vi "ResetHint.vi"(8 "No Error":errorcluster, 11 "Hint Name":T1) -> (0 "error out":errorcluster)   [LabVIEW 2024, in "SDL3.lvlib" / "Hints.lvlib"]
doc: "<B>Summary</B>\nReset a hint to the default value.\n\n<B>Remarks</B>\nThis will reset a hint to the value of the environment variable, or NULL if the environment isn't set. Callbacks will be called normally with this change."
uses:
  Hints.lvlib
  Lib/SDL3.dll
  HintName--combobox.ctl
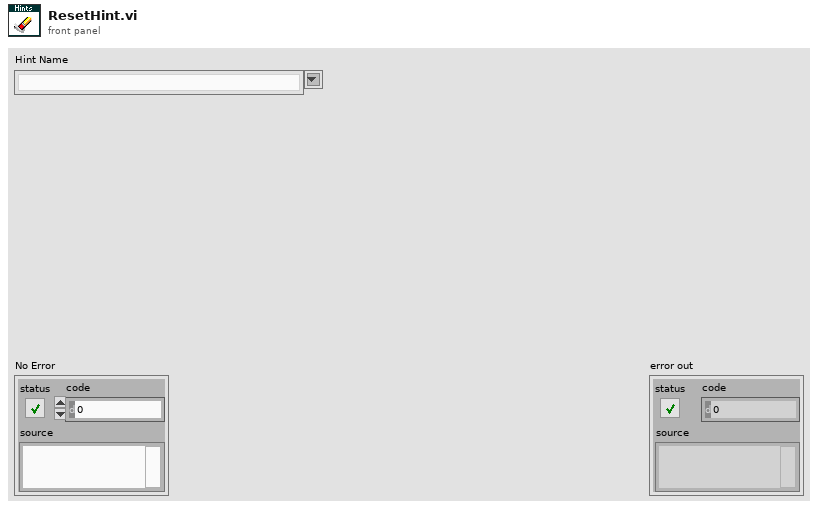
[diagram p1: front panel]
types:
  T1 = typedef "SDL3.lvlib/Hints.lvlib/HintName--combobox.ctl" = string
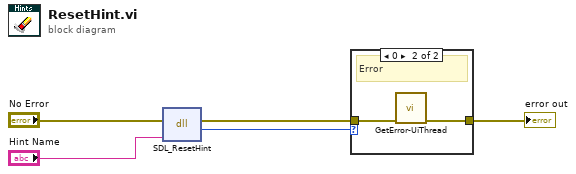
[diagram p0: block diagram]
diagram:
  n1 = dll-call lib="C:/Users/Thomas/Documents/Projects/LV-SDL3/Sources/SDL3/Lib/SDL3.*" fn="SDL_ResetHint"(error in="No Error", "name"="Hint Name") -> (error out=w3:errorcluster, "return type"=w1:i32)  [unwired: 3 in, 1 out]
  n2 = case shown="0" w1 {
    tunnel: w3 -> [w6 w8]
    tunnel: [w6 w7] -> w2
    frame Default {
      # "Ok"
    }
    frame 0 {
      # "Error"
      n3 = call "GetError-UiThread.vi"("No Error"=w8) -> ("error out"=w7:errorcluster)  [unwired: 10 in]
    }
  }
  "error out" <- w2
